vi "Prompt for Step--UI Interlocks.vi"(8 "error in (no error)":errorcluster, 10 "Control Refs":refnum<vi>[](array[refnum]), 11 "Mouse Action in":refnum<class "Mouse Action.lvclass">) -> (0 "error out":errorcluster, 2 "Step Valid?":bool, 3 "Mouse Action out":refnum<class "Mouse Action.lvclass">)   [LabVIEW 2020, in "MacroAssert.lvlib" / "Mouse Action.lvclass"]
uses:
  Mouse Action.lvclass
  Action Step/Action Step.lvclass
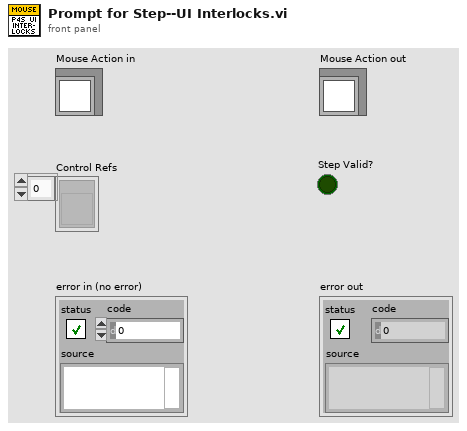
[diagram p1: front panel]
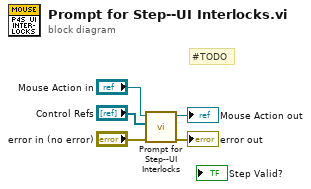
[diagram p0: block diagram]
diagram:
  # "#TODO"
  n1 = call-parent "Prompt for Step--UI Interlocks.vi"("error in (no error)"="error in (no error)", "Control Refs"="Control Refs", "Step in"="Mouse Action in") -> ("error out"=→"error out":errorcluster, "Step out"=→"Mouse Action out":refnum<class "Mouse Action.lvclass">)  [unwired: 6 in, 1 out]
